vi "LOC subConvertStringListTo2DArrayOfStrings.vi"(1 "InputString":string) -> (0 "OutputArray":string[][](array[string]))   [LabVIEW 2020, in "Localization_Tools.lvlib"]
uses:
  Localization_Tools.lvlib
panel:
  # "VI Name: LOC subConvert2DArrayOfStringsToStringList.vi\nDescription: Converts a list of strings to a 2D array of strings."
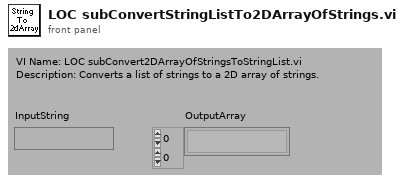
[diagram p1: front panel]
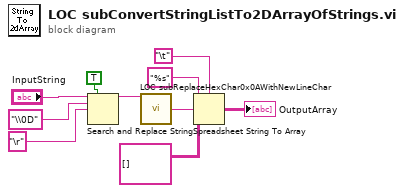
[diagram p0: block diagram]
diagram:
  n1 = Search and Replace String(replace all?=TRUE ("replace all? (F)"), input string="InputString", search string="\\0D" ("replace string (\"\")"), replace string="\r" ("replace string (\"\")")) -> (result string=w2:string)  [unwired: 4 in, 3 out]
  n2 = call "LOC subReplaceHexChar0x0AWithNewLineChar.vi"("InputString"=w2) -> ("OutputString"=w1:string)
  n3 = Spreadsheet String To Array(delimiter (Tab)="\t", format string="%s" ("delimiter (Tab)"), spreadsheet string=w1, array type (2D Dbl)=string[][] []) -> (array=→"OutputArray":string[][])
